vi "coercion-dot-consistency.vi"() -> ()   [LabVIEW 2025]
panel:
  in  "Enum":enum16{""}(ring)
  in  "dimension size":u32
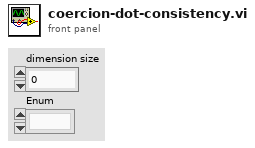
[diagram p1: front panel]
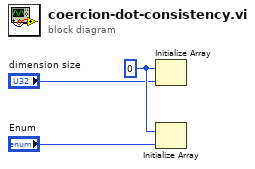
[diagram p0: block diagram]
diagram:
  w2 = 0 ("element")
  n1 = Initialize Array(w2, "dimension size") -> ()  [unwired: 1 out]
  n2 = Initialize Array(w2, "Enum") -> ()  [unwired: 1 out]
